vi "Read File.vi"(8 "error in (no error)":errorcluster, 10 "file path (use dialog)":path, 11 "Channel in":refnum<class "Channel.lvclass">) -> (0 "error out":errorcluster, 3 "Channel out":refnum<class "Channel.lvclass">)   [LabVIEW 2018, in "Channel.lvclass"]
uses:
  Channel.lvclass
  Channel.lvclass/Channel.ctl
  File interpreter/File interpreter.lvclass
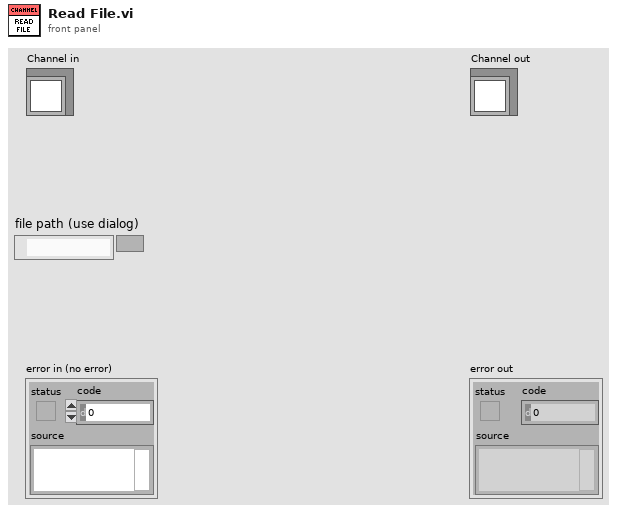
[diagram p1: front panel]
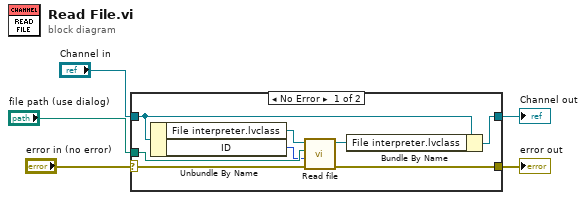
[diagram p0: block diagram]
diagram:
  n1 = case shown="No Error" "error in (no error)" {
    selector: "error in (no error)" -> [w10 w15]
    tunnel: [w11 w15] -> w4
    tunnel: [w12 w14] -> w2
    tunnel: "Channel in" -> [w13 w14]
    tunnel: "file path (use dialog)" -> [w7 _]
    frame No Error {
      n2 = Unbundle By Name(w13) -> ("File interpreter.lvclass"=w9:refnum<class "File interpreter.lvclass">, "ID"=w6:u16)
      n3 = call "Read file.vi"("error in (no error)"=w10, "Channel ID"=w6, "file path (use dialog)"=w7, "File interpreter in"=w9) -> ("error out"=w11:errorcluster, "File interpreter out"=w8:refnum<class "File interpreter.lvclass">)  [unwired: 6 in]
      n4 = Bundle By Name(cluster=w13, "File interpreter.lvclass"=w8) -> (w12:refnum<class "Channel.lvclass">)
    }
    frame Error {
    }
  }
  "error out" <- w4
  "Channel out" <- w2
